vi "Ctor.vi"(8 "error in (no error)":errorcluster, 11 "Websocket Client in":refnum<class "Websocket Client.lvclass">) -> (0 "error out":errorcluster, 3 "Websocket Client out":refnum<class "Websocket Client.lvclass">)   [LabVIEW 2020, in "Stream-Websocket.lvlib" / "Websocket Client.lvclass"]
uses:
  Websocket Client.lvclass
  Websocket Client.lvclass/Websocket Client.ctl
  WebsocketStream/WebsocketStream.lvclass
  Ref Data.ctl
  <vilib>/IlluminatedG/lv-stream/Connection/Connection.lvclass
  Client Command.ctl
  Stream-Websocket.lvlib
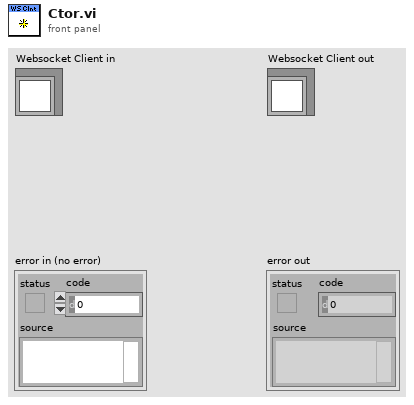
[diagram p1: front panel]
types:
  T1 = typedef "Stream-Websocket.lvlib/Client Command.ctl" = enum16{"Connect", "Close", "Shutdown", "Reconnect"}
  T2 = typedef "Stream-Websocket.lvlib/Websocket Client.lvclass/Ref Data.ctl" = cluster{"TCP Connection":refnum<k5>, "WS Stream":refnum<class "WebsocketStream.lvclass">, "Connection Loop":refnum<vi>, "Timeout ms":i32, "Server Connection":bool}
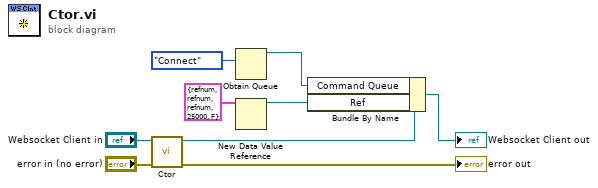
[diagram p0: block diagram]
diagram:
  n1 = call-parent "Ctor.vi"("error in (no error)"="error in (no error)", "Connection in"="Websocket Client in") -> ("error out"=→"error out":errorcluster, "Connection out"=w6:refnum<class "Websocket Client.lvclass">)  [unwired: 8 in]
  n2 = Obtain Queue(element data type=Client_Command."Connect" ("Command")) -> (queue out=w1:refnum<queue>)  [unwired: 4 in, 2 out]
  n3 = New Data Value Reference(data value=T2 {"TCP Connection"=refnum, "WS Stream"=refnum, "Connection Loop"=refnum, "Timeout ms"=25000, "Server Connection"=FALSE} ("Ref Data")) -> (data value reference=w5:refnum<data-value>)  [unwired: 1 in, 1 out]
  n4 = Bundle By Name(cluster=w6, "Command Queue"=w1, "Ref"=w5) -> (→"Websocket Client out":refnum<class "Websocket Client.lvclass">)
